vi "MIMO_TX.vi"() -> ()   [LabVIEW 2012]
uses:
  Synchronizer/Synchronizer.lvclass
  <instrlib>/niUSRP/niUSRP Write Tx Data (2D CDB).vi
  Transport Layer/UDP Tx.lvclass
panel:
  in  "UDP Listener":cluster{"Timeout":u16, "Local Port":u16}={"Timeout"=1, "Local Port"=1234}
  in  "ZC-Generation options":T1={"Sequence length"=64, "Sequence Root"=25, "# of subcarriers"=31, "Amplitude"=8.0, "Decimation Factor"=8, "Threshold"=20.0} {"Decimation Factor" min=1 max=8 step=1}
  out "Tx Queue":dbl[](graph)=[0.0, 391.0, 895.0, 0.0, 0.0, 0.0, 0.0, 391.0, 895.0, 0.0, 0.0, 0.0, 0.0, 391.0, 895.0, 0.0, 0.0, 0.0, 0.0, 0.0, 0.0, 0.0, 0.0, 391.0, 895.0, 0.0, 0.0, 0.0, 0.0, 0.0, 391.0, 895.0, 0.0, 0.0, 0.0, 0.0, 391.0, 895.0, 0.0, 0.0, 0.0, 0.0, 0.0, 0.0, 391.0, 895.0, 0.0, 0.0, 0.0, 0.0, 391.0, 895.0, 0.0, 0.0, 0.0, 0.0, 391.0, 895.0, 0.0, 0.0, 0.0, 0.0, 0.0, 391.0, 895.0, 0.0, 0.0, 0.0, 0.0, 391.0, 895.0, 0.0, 0.0, 0.0, 0.0, 0.0, 0.0, 0.0, 391.0, 895.0, 0.0, 0.0, 0.0, 0.0, 0.0, 0.0, 391.0, 895.0, 0.0, 0.0, 0.0, 0.0, 391.0, 895.0, 0.0, 0.0, 0.0, 0.0, 0.0, 0.0, 391.0, 895.0, 0.0, 0.0, 0.0, 0.0, 391.0, 895.0, 0.0, 0.0, 0.0, 0.0, 391.0, 895.0, 0.0, 0.0, 0.0, 0.0, 391.0, 895.0, 0.0, 0.0, 0.0, 0.0, 0.0, 0.0, 391.0, 895.0, 0.0, 0.0, 0.0, 0.0, 0.0, 0.0, 391.0, 895.0, 0.0, 0.0, 0.0, 0.0, 0.0, 391.0, 895.0, 0.0, 0.0, 0.0, 0.0, 0.0, 391.0, 895.0, 0.0, 0.0, 0.0, 0.0, 0.0, 0.0, 391.0, 895.0, 0.0, 0.0, 0.0, 0.0, 391.0, 895.0, 0.0, 0.0, 0.0, 0.0, 391.0, 895.0, 0.0, 0.0, 0.0, 0.0, 391.0, 895.0, 0.0, 0.0, 0.0, 0.0, 0.0, 0.0, 0.0, 0.0, 391.0, 895.0, 0.0, 0.0, 0.0, 0.0, 391.0, 895.0, 0.0, 0.0, 0.0, 0.0, 0.0, 391.0, 895.0, 0.0, 0.0, 0.0, 0.0, 391.0, 895.0, 0.0, 0.0, 0.0, 0.0, 0.0, 0.0, 0.0, 391.0, 895.0, 0.0, 0.0, 0.0, 0.0, 391.0, 895.0, 0.0, 0.0, 0.0, 0.0, 391.0, 895.0, 0.0, 0.0, 0.0, 0.0, 391.0, 895.0, 0.0, 0.0, 0.0, 0.0, 0.0, 0.0, 391.0, 895.0, 0.0, 0.0, 0.0, 0.0, 0.0, 0.0, 391.0, 895.0, 0.0, 0.0, 0.0, 0.0, 0.0, 391.0, 895.0, 0.0, 0.0, 0.0, 0.0, 391.0, 895.0, 0.0, 0.0, 0.0, 0.0, 0.0, 0.0, 391.0, 895.0, 0.0, 0.0, 0.0, 0.0, 0.0, 391.0, 895.0, 0.0, 0.0, 0.0, 0.0, 391.0, 895.0, 0.0, 0.0, 0.0, 0.0, 391.0, 895.0, 0.0, 0.0, 0.0, 0.0, 0.0, 391.0, 895.0, 0.0, 0.0, 0.0, 0.0, 0.0, 0.0, 0.0, 391.0, 895.0, 0.0, 0.0, 0.0, 0.0, 0.0, 391.0, 895.0, 0.0, 0.0, 0.0, 0.0, 391.0, 895.0, 0.0, 0.0, 0.0, 0.0, 0.0, 0.0, 391.0, 895.0, 0.0, 0.0, 0.0, 0.0, 391.0, 895.0, 0.0, 0.0, 0.0, 0.0, 0.0, 391.0, 895.0, 0.0, 0.0, 0.0, 0.0, 391.0, 895.0, 0.0, 0.0, 0.0, 0.0, 391.0, 895.0, 0.0, 0.0, 0.0, 0.0, 0.0, 0.0, 0.0, 0.0, 391.0, 895.0, 0.0, 0.0, 0.0, 0.0, 0.0, 391.0, 895.0, 0.0, 0.0, 0.0, 0.0, 391.0, 895.0, 0.0, 0.0, 0.0, 0.0, 0.0, 0.0, 391.0, 895.0, 0.0, 0.0, 0.0, 0.0, 391.0, 895.0, 0.0, 0.0, 0.0, 0.0, 391.0, 895.0, 0.0, 0.0, 0.0, 0.0, 0.0, 391.0, 895.0, 0.0, 0.0, 0.0, 0.0, 0.0, 391.0, 895.0, 0.0, 0.0, 0.0, 0.0, 0.0, 0.0, 391.0, 895.0, 0.0, 0.0, 0.0, 0.0, 0.0, 0.0, 391.0, 895.0, 0.0, 0.0, 0.0, 0.0, 391.0, 895.0, 0.0, 0.0, 0.0, 0.0, 0.0, 0.0, 391.0, 895.0, 0.0, 0.0, 0.0, 0.0, 391.0, 895.0, 0.0, 0.0, 0.0, 0.0, 391.0, 895.0, 0.0, 0.0, 0.0, 0.0, 391.0, 895.0, 0.0, 0.0, 0.0, 0.0, 0.0, 0.0, 391.0, 895.0, 0.0, 0.0, 0.0, 0.0, 0.0, 0.0, 391.0, 895.0, 0.0, 0.0, 0.0, 0.0, 0.0, 391.0, 895.0, 0.0, 0.0, 0.0, 0.0, 0.0, 391.0, 895.0, 0.0, 0.0, 0.0, 0.0, 0.0, 0.0, 391.0, 895.0, 0.0, 0.0, 0.0, 0.0, 391.0, 895.0, 0.0]
  out "Link Occupation":dbl[](graph)=[40.54831201730021, 40.17426097626925, 39.569960582090154, 38.95955614352541, 39.353087013662034, 39.75059294309296, 40.15211408393228, 39.77406104357438, 39.165718225832705, 38.55123053114415, 38.940636900145606, 39.33397666681374, 39.73128956243812, 39.34898576933785, 38.73634926195743, 38.1175245070277, 38.50255000709869, 38.89146465363504, 39.284307730944484, 39.68111892014594, 40.08193830317772, 40.48680636684618, 40.895764006915336, 40.525222581941094, 39.924467254485954, 39.31764369139995, 39.7147916074747, 40.115951118661314, 40.52116274612254, 40.9304674203258, 40.560276534880956, 39.95987528775854, 39.35340938157429, 39.75091856724676, 40.15244299721895, 40.55802322951409, 40.184070281535796, 39.57986897124828, 38.969564617422506, 39.36319658325506, 39.76080462955056, 40.162428918737945, 40.568110018927214, 40.97788890800729, 40.60817702748852, 40.008259623725785, 39.40228244820786, 39.800285301220065, 40.20230838507077, 40.6083923081523, 40.234948138746105, 39.631260746208184, 39.02147550122039, 39.415631819414536, 39.813769514560136, 40.215928802586, 39.83852035534581, 39.230828641763445, 38.61699862804388, 39.007069321256445, 39.40108012248126, 39.799070830789155, 40.20108164726177, 39.823523228755676, 39.21568002904614, 38.601696999036506, 38.99161313033991, 39.385467808424146, 39.78330081659005, 39.40152238969333, 38.78941655524579, 38.17112783358161, 38.556694781395564, 38.946156344844006, 39.339551863478796, 39.73692107422101, 40.13830411537476, 40.54374153068157, 40.16964432311911, 39.565297296079905, 38.95484575361606, 39.34832904405663, 39.74578691318851, 40.147259508271226, 40.55278738209215, 40.962411497062774, 40.59254327905972, 39.99246795864618, 39.38633127135978, 39.78417300137352, 40.186033334720726, 40.59195286335427, 40.21834263895012, 39.61448751409103, 39.00453284251619, 39.39851802274363, 39.796482851256194, 40.198467526521405, 40.60451265305193, 41.014659245507, 40.64531878253873, 40.04577654801892, 39.44017833133224, 39.83856397104267, 40.24097370812391, 40.64744819002415, 40.27439852447525, 39.671109620682074, 39.061726889577855, 39.45628978745238, 39.85483816914382, 40.257412292064465, 39.880422869970516, 39.27315441411163, 38.65975193344609, 39.050254478228375, 39.444701493159975, 39.843132821373715, 39.46195875816168, 38.8504633920825, 38.232791305133844, 38.618981116296816, 39.00907183464325, 39.40310286327601, 39.8011140033091, 40.203145457887985, 39.82560788595387, 39.21778574338775, 38.603823983219954, 38.99376159921207, 39.38763797900209, 39.78549290808292, 40.18736657382114, 40.5932995695163, 40.21970294820469, 39.615861563843126, 39.00592077155871, 39.39991997127143, 39.79789896088023, 40.199897940283066, 40.60595751543744, 40.232488752165445, 39.628776517338835, 39.01896617913014, 39.4130971506365, 39.811209243067175, 40.21334266976482, 40.619538050267494, 40.24620646411499, 39.64263279203534, 39.032962416197314, 39.42723476383567, 39.82548966044007, 40.22776733377785, 40.63410841795742, 41.04455395753275, 40.675515461352624, 40.07627824379053, 39.47098812504094, 39.869684974788825, 40.272409065443256, 40.67920107620531, 40.30647214688046, 39.70350721907117, 39.09445173643552, 39.48934518831871, 39.888227462948194, 40.291138851462826, 39.914490101686035, 39.30756575927882, 38.69451086795841, 39.0853645130893, 39.48016617483768, 39.87895573215927, 39.49814351653093, 38.887013653061544, 38.269710760668225, 38.65627349562447, 39.04674090467118, 39.44115242896079, 39.839547908041204, 40.241967583880005, 40.6484521049293, 41.059042530231615, 40.69015038327067, 40.091060993202696, 39.485920195154236, 39.88476787389317, 40.28764431706381, 40.69459021925637, 40.322016735820924, 39.71920882406154, 39.110311943496505, 39.50536559949142, 39.90440969645598, 40.30748454187473, 40.71463085037851, 40.342259797560466, 39.73965636117219, 39.13096602138605, 39.526228304430354, 39.925483135788234, 40.32877084423054, 39.952502215592816, 39.34596183393214, 38.733294781749635, 39.12454018358549, 39.51973755917726, 39.91892682745178, 40.32214831055735, 40.72944273793672, 41.14085125044113, 40.772785454189375, 40.174530761807446, 39.570233092734796, 39.96993241690384, 40.37366910798367, 40.781483947458256, 40.4097881784491, 39.80786684691828, 39.19986550193766, 39.59582373933097, 39.99578155487976, 40.399779348363396, 40.02422797734317, 39.418412098326435, 38.8064768669964, 39.19846148181455, 39.59440553718641, 39.99434902746102, 39.61470240067411, 39.00474989967082, 38.38863626229376, 38.77640026494319, 39.168081075700194, 39.563718258283025, 39.96335177604346, 40.367021996003494, 39.99113974263621, 39.38498963902647, 38.772716807097446, 39.16436041120954, 39.55996001132277, 39.9595555669927, 40.363187441406765, 40.77089640546138, 40.399093691583566, 39.7970643349329, 39.1889538736696, 39.58480189259555, 39.98464837635914, 40.388533713494084, 40.79649870049907, 40.424954595662044, 39.823186460264694, 39.21533985885323, 39.611454402882046, 40.01157010392126, 40.41572737769824, 40.04033709788342, 39.43468393725598, 38.82291306793534, 39.21506370498519, 39.611175459581, 40.01128834301111, 40.41544277071829, 40.82367956638212, 40.452410015745926, 39.85091920782417, 39.24335273517593, 39.639750237551446, 40.04015175510247, 40.444597732426736, 40.85312902265327, 40.48215694127234, 39.880966607345805, 39.27370364378364, 39.67040772099358, 40.071118910094526, 40.47587768696417, 40.10109498603082, 39.49605554144527, 38.88490458731846, 39.277681401331776, 39.67442565791089, 40.07517743223322, 39.69634725397936, 39.087219448464005, 38.47193883683233, 38.86054427962861, 39.25307502992789, 39.6495707373009, 40.050071451819086, 39.67098767780347, 39.061603714952994, 38.44606435853838, 38.83440844296806, 39.226675194917235, 39.622904237290136, 40.023135593222364, 40.4274096901236, 40.835767363761214, 40.464619912088445, 39.863252436452974, 39.25581054187169, 39.652333880678476, 40.05286250573584, 40.45743687448064, 40.86609785301075, 40.49525676991626, 39.894198757491175, 39.28706945201129, 39.683908537385136, 40.08475609836883, 40.489652624614976, 40.11500906446599, 39.51011016612726, 38.899101177906324, 39.29202139182457, 39.688910496792495, 40.08980858261868, 40.494756144059274, 40.903794084908355, 40.533333771833036, 39.932660375588924, 39.325919571301945, 39.72315108212318, 40.12439503244766, 40.52969195196733, 40.15545282946836, 39.55096245400844, 38.940366115160046, 39.33370314662631, 39.731013279420516, 40.132336645879306, 40.53771378371647, 40.16355568982103, 39.559147161435384, 38.94863349639938, 39.34205403676705, 39.73944852198692, 40.140857092916086, 39.762690345578214, 39.15423267230123, 38.53962896192043, 38.92891814335397, 39.32213953874138, 39.71933286741554, 39.33690829961807, 38.72414979759401, 38.10520181575153, 38.490102844193466, 38.87889176181158, 39.27160784021372, 39.66829074769063, 40.06898055322286, 40.473717730528136, 40.88254316214963, 40.51186819328887, 39.91097797301906, 39.30401815456471, 39.70102843895425, 40.10204892823662, 40.50712012953194, 40.91628295912317, 40.54594879629244, 39.94540282453782, 39.338790731856385, 39.73615225440039, 40.13752752969736, 40.542957100704406, 40.16885196960682, 39.56449693899679, 38.95403731211797, 39.347512436482795, 39.74496205705333, 40.14642632025589, 40.551945778036256, 40.96156139195581, 40.59168458703248, 39.9916005929621, 39.385455144406166, 39.78328802465269, 40.1851394188411, 40.59104991802132, 40.21743057295724, 39.613566235310344, 39.003602257889234, 39.39757803827195, 39.79553337199187, 40.19750845655745, 39.81991394521596, 39.21203428809693, 38.598014432421145, 38.98789336608196, 39.38171047078986, 39.779505526050364, 40.181318713182186, 39.803560669079324, 39.19551582735286, 38.58132911853824, 38.971039513674995, 39.36468637744949, 39.7623094721712, 40.16394896178909, 39.78601546565196, 39.17779339964844, 38.56342767641257, 38.95295724890159, 39.34642146353696, 39.74386006417875, 40.14531319614015, 40.55082141024258, 40.176795716615075, 39.57252092587381, 38.96214234936748, 39.35569934279544, 39.753231659389336, 40.15477945392862, 40.560383286796586, 40.97008412807736, 40.600293411397686, 40.000296375149176, 39.39423876277694, 39.79216036644136, 40.194101380243794, 40.60010240428666, 40.22657449847779, 39.62280252371494, 39.012931842136304, 39.40700186074374, 39.80505238458964, 40.20712362079761, 40.61325618262385, 41.02349109355944, 40.654239841177564, 40.054787718361176, 39.449280523597146, 39.84775810464358, 40.25026071176119, 40.65682900177898, 40.28387409190437, 39.68068090091351, 39.07139484940758, 39.466055403442006, 39.8647024277192, 40.267376189615355, 39.89048741295122, 39.28332061914264, 38.67002082741681, 39.06062709840082, 39.45517888727356, 39.85371604775107, 39.47264888581557, 38.861261500823815, 38.243698485680625, 38.62999847038447, 39.02020047513583, 39.41434391427862, 39.812468600281434, 40.21461474775902, 39.837193027237745, 39.229487906300754, 38.61564434979874, 39.005701363433076, 39.3996983469021, 39.797675097880905, 40.19967181604132, 40.60572910711244, 40.23225803668564, 39.62854347139964, 39.01873077919156, 39.412859372920764, 39.81096906355633, 40.213100064198315, 40.61929299413971, 40.24595893267279, 39.642382760275545, 39.03270985886419, 39.42697965541837, 39.82523197517007, 40.22750704562633, 40.63384550063266, 40.26065843418082, 39.657230741596784, 39.04770781979473, 39.44212911090377, 39.840534455458354, 40.24296409642258, 40.64945868325513, 41.06005927601529, 40.69117739921377, 40.09209838304422, 39.486968063681026, 39.88582632695053, 40.28871346156619, 40.69567016319817, 40.32310758828739, 39.72031069523979, 39.111424944686654]
  out "UDP Received Packet":bool
  out "Tx Buffer size":i32
  out "Ok?":bool=TRUE
  in  "Send Message":bool
  in  "Send Message":string="The quick brown fox jumps over the lazy dog"
  in  "System options":T2={"Samples per symbol"=6, "Roll-Off"=0.75, "Filter length (symbols)"=3, "Symbols/Pilots"=6, "Modulation Type"=enum."16-QAM", "Payload Symbols"=1008} {"Payload Symbols" min=32 max=8192 step=16; "Symbols/Pilots" min=6 max=16 step=2; "Filter length (symbols)" min=1 max=9 step=2; "Roll-Off" min=0.0 max=1.0 step=0.01; "Samples per symbol" min=2 max=32 step=2}
  in  "Tx Parameters":T3={"IQ rate (Hz)"=500000.0, "Carrier frequency [Hz]"=1187500000.0, "Gain [dB]"=13.0, "Tx device name"="192.168.10.2; 192.168.10.3;"} {"Gain [dB]" format="%#_6f"; "Carrier frequency [Hz]" format="%#_6p"; "IQ rate (Hz)" format="%#_6p"}
  in  "stop":bool
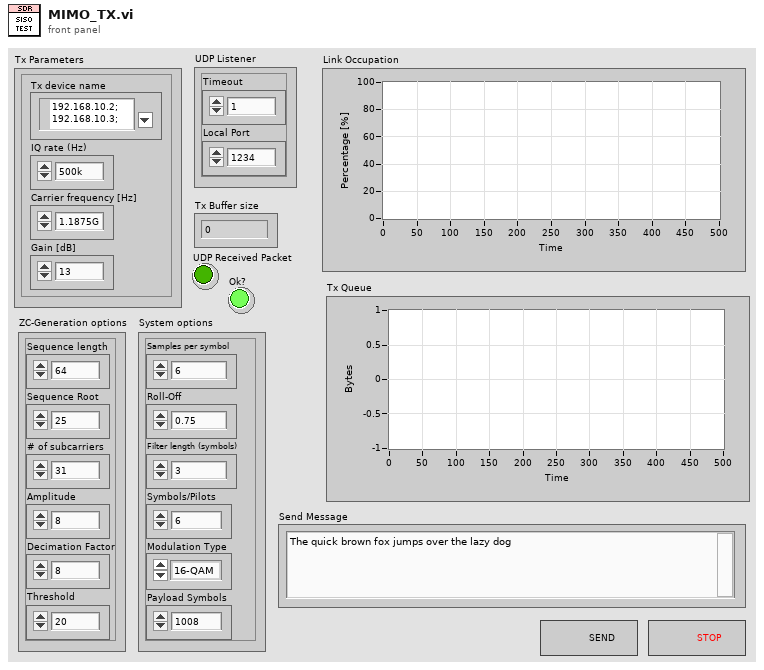
[diagram p1: front panel]
types:
  T1 = cluster{"Sequence length":i32, "Sequence Root":i32, "# of subcarriers":i32, "Amplitude":dbl, "Decimation Factor":u8, "Threshold":dbl}
  T2 = cluster{"Samples per symbol":i32, "Roll-Off":dbl, "Filter length (symbols)":i32, "Symbols/Pilots":i32, "Modulation Type":enum16{"BPSK", "4-QAM", "16-QAM", "64-QAM"}, "Payload Symbols":i32}
  T3 = cluster{"IQ rate (Hz)":dbl, "Carrier frequency [Hz]":dbl, "Gain [dB]":dbl, "Tx device name":refnum<k15>}
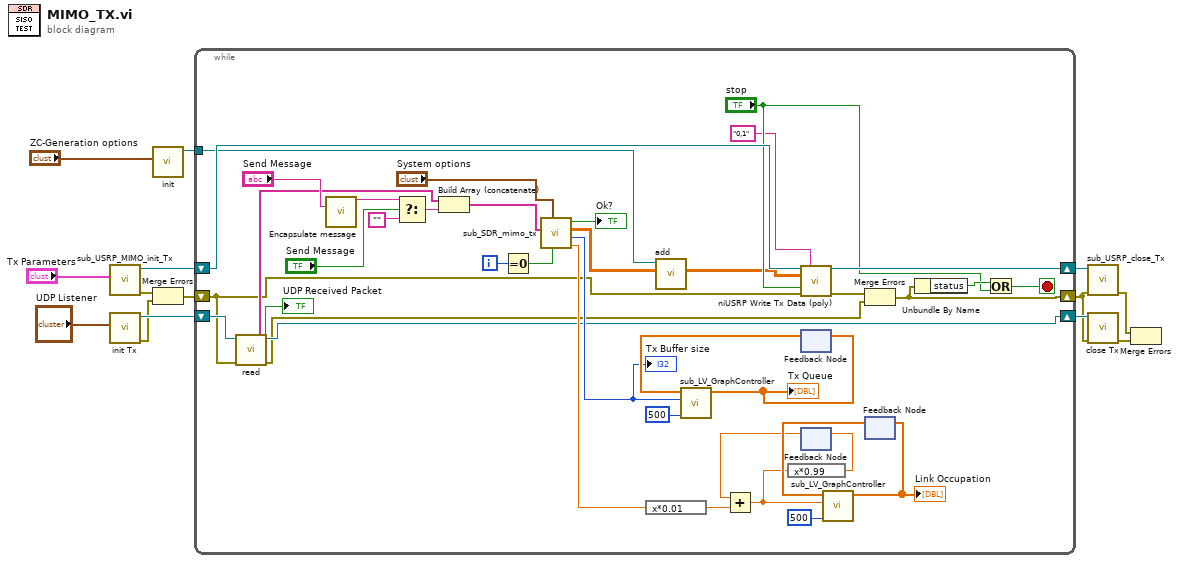
[diagram p0: block diagram]
diagram:
  n1 = call "sub_USRP_MIMO_init_Tx.vi"("Tx Parameters"="Tx Parameters") -> ("Error out"=w6:errorcluster, "Tx Session handle out"=w14:refnum<k15>)  [unwired: 9 in]
  n2 = call "init Tx.vi"("Cluster"="UDP Listener") -> ("error out"=w5:errorcluster, "UDP Tx.lvclass"=w9:refnum<class "UDP Tx.lvclass">)  [unwired: 9 in]
  n3 = call "init.vi"("ZC-Generation options"="ZC-Generation options") -> ("Synchronizer out"=w10:refnum<class "Synchronizer.lvclass">)  [unwired: 9 in, 1 out]
  n4 = Merge Errors(w6, w5) -> (w3:errorcluster)
  n5 = while {
    shift-right: [w49] -> w12
    shift-left: w14 -> [w50]
    shift-right: [w16] -> w4
    shift-left: w3 -> [w15]
    tunnel: w10 -> [w23]
    shift-right: [w19] -> w7
    shift-left: w9 -> [w20]
    i -> [w53]
    stop <- w51 stop-if-true
    n6 = call "read.vi"("error in (no error)"=w15, "UDP Tx in"=w20) -> ("error out"=w17:errorcluster, "Received Packet"=→"UDP Received Packet":bool, "Received data"=w22:string[], "UDP Tx out"=w19:refnum<class "UDP Tx.lvclass">)  [unwired: 6 in]
    n7 = call "Encapsulate message"("Message"="Send Message") -> ("Result"=w46:string)  [unwired: 13 in, 1 out]
    n8 = Select(t=w46, s="Send Message", f="") -> (s? t:f=w39:string)
    n9 = Build Array (concatenate)(w22, w39) -> (w26:string[])
    n10 = Equal To 0?(x=w53) -> (x = 0?=w43:bool)
    n11 = call "sub_SDR_mimo_tx.vi"("Init Tx Buffer"=w43, "System options"="System options", "Packets"=w26) -> ("Link occupation [%]"=w32:dbl, "Tx Buffer size"=w28:i32, "Tx Frame"=w24:cdb[][], "Ok?"=→"Ok?":bool)  [unwired: 5 in]
    "Tx Buffer size" <- w28
    n12 = expression code="x*0.01"(w32) -> (w33:dbl)
    n13 = call-dynamic "add.vi"("Input Frame"=w24, "Synchronizer in"=w23) -> ("Output Frame"=w25:cdb[][])  [unwired: 7 in, 2 out]
    n14 = call-poly <instrlib>:"niUSRP Write Tx Data (poly).vi"("session handle"=w50, "channel list"="0,1", "data"=w25, "end of data?"="stop", "error in (no error)"=w15) -> ("session handle out"=w49:refnum<k15>, "error out"=w18:errorcluster)  [unwired: 9 in]
    n15 = feedback #1() -> (w30:dbl[])  [unwired: 1 in]
    n16 = call "sub_LV_GraphController.vi"("Number of samples"=500, "Input sample"=w28, "Prev. data"=w30) -> ("Graph data"=w27:dbl[])  [unwired: 8 in]
    "Tx Queue" <- w27
    n17 = feedback-in #1(w27) -> ()
    n18 = feedback #2() -> (w34:dbl)  [unwired: 1 in]
    n19 = Add(x=w34, y=w33) -> (x+y=w31:dbl)
    n20 = expression code="x*0.99"(w31) -> (w35:dbl)
    n21 = feedback-in #2(w35) -> ()
    n22 = Merge Errors(w18, w17) -> (w16:errorcluster)
    n23 = feedback #3() -> (w38:dbl[])  [unwired: 1 in]
    n24 = call "sub_LV_GraphController.vi"("Number of samples"=500, "Input sample"=w31, "Prev. data"=w38) -> ("Graph data"=w36:dbl[])  [unwired: 8 in]
    "Link Occupation" <- w36
    n25 = feedback-in #3(w36) -> ()
    n26 = Unbundle By Name(w16) -> ("status"=w52:bool)
    n27 = Or(x=w52, y="stop") -> (x .or. y?=w51:bool)
  }
  n28 = call "sub_USRP_close_Tx.vi"("Error in"=w4, "Tx Session handle"=w12) -> ("Error out"=w1:errorcluster)  [unwired: 9 in]
  n29 = call "close Tx.vi"("error in (no error)"=w4, "UDP Tx in"=w7) -> ("error out"=w2:errorcluster)  [unwired: 9 in]
  n30 = Merge Errors(w1, w2) -> ()  [unwired: 1 out]
